vi "Begin.vi"(8 "error in":errorcluster) -> (0 "error out":errorcluster)   [LabVIEW 2015]
doc: "Called before other user functions, this VI is expected to open initial I/O refnums, load in file data, and do all program initialization. Notice that the <B>error out</B> terminal is simply used for data flow. Wiring it to other structures or subVIs ensures that this VI runs first."
uses:
  <vilib>/Rock Robotics/SystemInterfaces/DIO/FPGA_DIOPWMChannel.ctl
  <vilib>/Rock Robotics/WPI/SafetyOutput/WPI_SafetyOutputConfigMenu.ctl
  <vilib>/Rock Robotics/WPI/DriverStation/WPI_DriverStationRobotMode2.ctl
  <vilib>/Rock Robotics/WPI/Joystick/WPI_JoystickDeviceEnum.ctl
  <vilib>/Rock Robotics/SystemInterfaces/DIO/FPGA_DIOChannel.ctl
  <vilib>/Rock Robotics/SystemInterfaces/DIO/FPGA_DIORelayChannel.ctl
  <vilib>/Rock Robotics/WPI/Encoder/WPI_EncoderType.ctl
  <vilib>/Rock Robotics/WPI/Relay/WPI_RelayDirection.ctl
  <vilib>/Rock Robotics/SystemInterfaces/spilib/spi_bus.ctl
  <vilib>/Rock Robotics/WPI/RobotDrive/WPI_RobotDriveOpen2MotorWithVictor.vi
  Robot Global Data.vi
  <vilib>/Rock Robotics/Network Tables/NT Write String Array.vi
  <vilib>/Rock Robotics/WPI/Counter/WPI_CounterDigitalInputToDigitalSource.vi
  <vilib>/Rock Robotics/WPI/MotorControl/WPI_MotorControlOpen Victor.vi
  <vilib>/Rock Robotics/WPI/Gyro/WPI_GyroXRS450_SPI_Open.vi
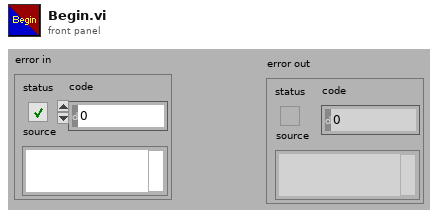
[diagram p1: front panel]
types:
  T1 = typedef "spi_bus.ctl" = enum16{"SPI On-Board, CS0", "SPI On-Board, CS1", "SPI On-Board, CS2", "SPI On-Board, CS3", "SPI MXP", "Invalid"}
  T2 = typedef "FPGA_DIOPWMChannel.ctl" = enum8{"PWM 0", "PWM 1", "PWM 2", "PWM 3", "PWM 4", "PWM 5", "PWM 6", "PWM 7", "PWM 8", "PWM 9", "PWM MXP 0", "PWM MXP 1", "PWM MXP 2", "PWM MXP 3", "PWM MXP 4", "PWM MXP 5", "PWM MXP 6", "PWM MXP 7", "PWM MXP 8", "PWM MXP 9", "Invalid"}
  T3 = typedef "WPI_RelayDirection.ctl" = enum16{"Both directions", "Forward only", "Reverse only"}
  T4 = typedef "FPGA_DIORelayChannel.ctl" = enum8{"Relay 0", "Relay 1", "Relay 2", "Relay 3", "Invalid"}
  T5 = typedef "FPGA_DIOChannel.ctl" = enum8{"DIO 0", "DIO 1", "DIO 2", "DIO 3", "DIO 4", "DIO 5", "DIO 6", "DIO 7", "DIO 8", "DIO 9", "DIO MXP 0", "DIO MXP 1", "DIO MXP 2", "DIO MXP 3", "DIO MXP 4", "DIO MXP 5", "DIO MXP 6", "DIO MXP 7", "DIO MXP 8", "DIO MXP 9", "DIO MXP 10", "DIO MXP 11", "DIO MXP 12", "DIO MXP 13", "DIO MXP 14", "DIO MXP 15", "Invalid"}
  T6 = typedef "WPI_EncoderType.ctl" = enum16{"1x", "2x", "4x"}
  T7 = typedef "WPI_JoystickDeviceEnum.ctl" = enum16{"USB 0", "USB 1", "USB 2", "USB 3", "USB 4", "USB 5"}
  T8 = typedef "WPI_SafetyOutputConfigMenu.ctl" = enum16{"Enable", "Disable"}
  T9 = typedef "WPI_DriverStationRobotMode2.ctl" = enum16{"Autonomous Disabled", "Autonomous Enabled", "Teleop Disabled", "Teleop Enabled", "Disconnected", "Finish", "Test Disabled", "Test Enabled", "Emergency Stopped"}
  T10 = typedef "WPI_MotorControlDeviceRef.ctl" = cluster{"DeviceStatus":errorcluster, "Type":T11, "PWM":cluster{"PWM Channel":T2, "DeadBand":T12}, "CAN":cluster{"Device Number":u8, "Control Mode":T13, "Semaphore":T14, "Max Vout":dbl, "TalonSRX Control Mode":T15}, "Invert":bool}
  T11 = typedef "WPI_MotorControlType.ctl" = enum16{"PWM", "CAN", "CANTalonSRX"}
  T12 = typedef "WPI_PWMDeadband.ctl" = cluster{"Name":string, "maxPositivePwm":i32, "minPositivePwm":i32, "centerPwm":i32, "maxNegativePwm":i32, "minNegativePwm":i32, "angularRange":u16}
  T13 = typedef "WPI_CANJaguar_ControlMode.ctl" = enum8{"Percent VBus", "Current", "Speed", "Position", "Voltage"}
  T14 = typedef "Semaphore RefNum" = refnum<k1>
  T15 = typedef "WPI_CANTalonSRX_APIControlMode.ctl" = enum8{"Percent VBus", "Speed", "Position", "Slave", "Unchanged / Invalid", "Voltage Compensation", "Current", "Motion Profile"}
  T16 = typedef "WPI_JoystickDevRef.ctl" = cluster{"Device":T7}
  T17 = typedef "WPI_RobotDriveDevRef.ctl" = cluster{"DevStatus":errorcluster, "Motors[]":T10[], "Square Inputs":bool, "Max Output":dbl}
  T18 = typedef "WPI_RelayDevRef.ctl" = cluster{"DevStatus":errorcluster, "Relay Channel":T4, "Relay Direction":T3}
  T19 = typedef "WPI_DigitalInputDevRef.ctl" = cluster{"DevStatus":errorcluster, "DIO Channel":T5}
  T20 = typedef "FPGA_CounterEncoderSourceConvertionLVSourceType.ctl" = cluster{"DevStatus":errorcluster, "AnalogTriggerMode?":bool, "DigitalMode":cluster{"DIO Channel":T21}, "AnalogTriggerMode":cluster{"AnalogTriggerIndex":T22, "OutputType":T23}}
  T21 = typedef "FPGA_DIODigitalSourceChannel.ctl" = enum8{"DIO 0", "DIO 1", "DIO 2", "DIO 3", "DIO 4", "DIO 5", "DIO 6", "DIO 7", "DIO 8", "DIO 9", "DIO MXP 0", "DIO MXP 1", "DIO MXP 2", "DIO MXP 3", "DIO MXP 4", "DIO MXP 5", "DIO MXP 6", "DIO MXP 7", "DIO MXP 8", "DIO MXP 9", "DIO MXP 10", "DIO MXP 11", "DIO MXP 12", "DIO MXP 13", "DIO MXP 14", "DIO MXP 15", "Disabled"}
  T22 = typedef "FPGA_AnalogTriggerIndex.ctl" = enum8{"Trig 0", "Trig 1", "Trig 2", "Trig 3", "Trig 4", "Trig 5", "Trig 6", "Trig 7", "Invalid"}
  T23 = typedef "FPGA_AnalogTriggerOutType.ctl" = enum16{"InWindow", "TriggerState", "Rising", "Falling"}
  T24 = typedef "WPI_EncoderDevRef.ctl" = cluster{"DevStatus":errorcluster, "EncoderIndex":T25, "CounterIndex":T26, "DistancePerCount":dbl, "Decoding Type":T6}
  T25 = typedef "FPGA_EncoderIdx.ctl" = enum8{"Enc 0", "Enc 1", "Enc 2", "Enc 3", "Enc 4", "Enc 5", "Enc 6", "Enc 7", "Invalid"}
  T26 = typedef "FPGA_CounterCtrSystemIndex.ctl" = enum8{"Ctr 0", "Ctr 1", "Ctr 2", "Ctr 3", "Ctr 4", "Ctr 5", "Ctr 6", "Ctr 7", "Invalid"}
  T27 = typedef "WPI_GyroDevRef.ctl" = cluster{"DevStatus":errorcluster, "Analog Channel":T28, "Offset":dbl, "Gain (VoltsPerDegree/Second)":dbl, "Gyro Type":enum16{"Analog", "XRS450"}, "Handle":i32, "SPI Bus":T1, "Device Found":bool, "Sample Rate":dbl, "Calibrate On Open":bool}
  T28 = typedef "FPGA_AIChannel.ctl" = enum8{"AI 0", "AI 1", "AI 2", "AI 3", "AI MXP 0", "AI MXP 1", "AI MXP 2", "AI MXP 3", "Invalid"}
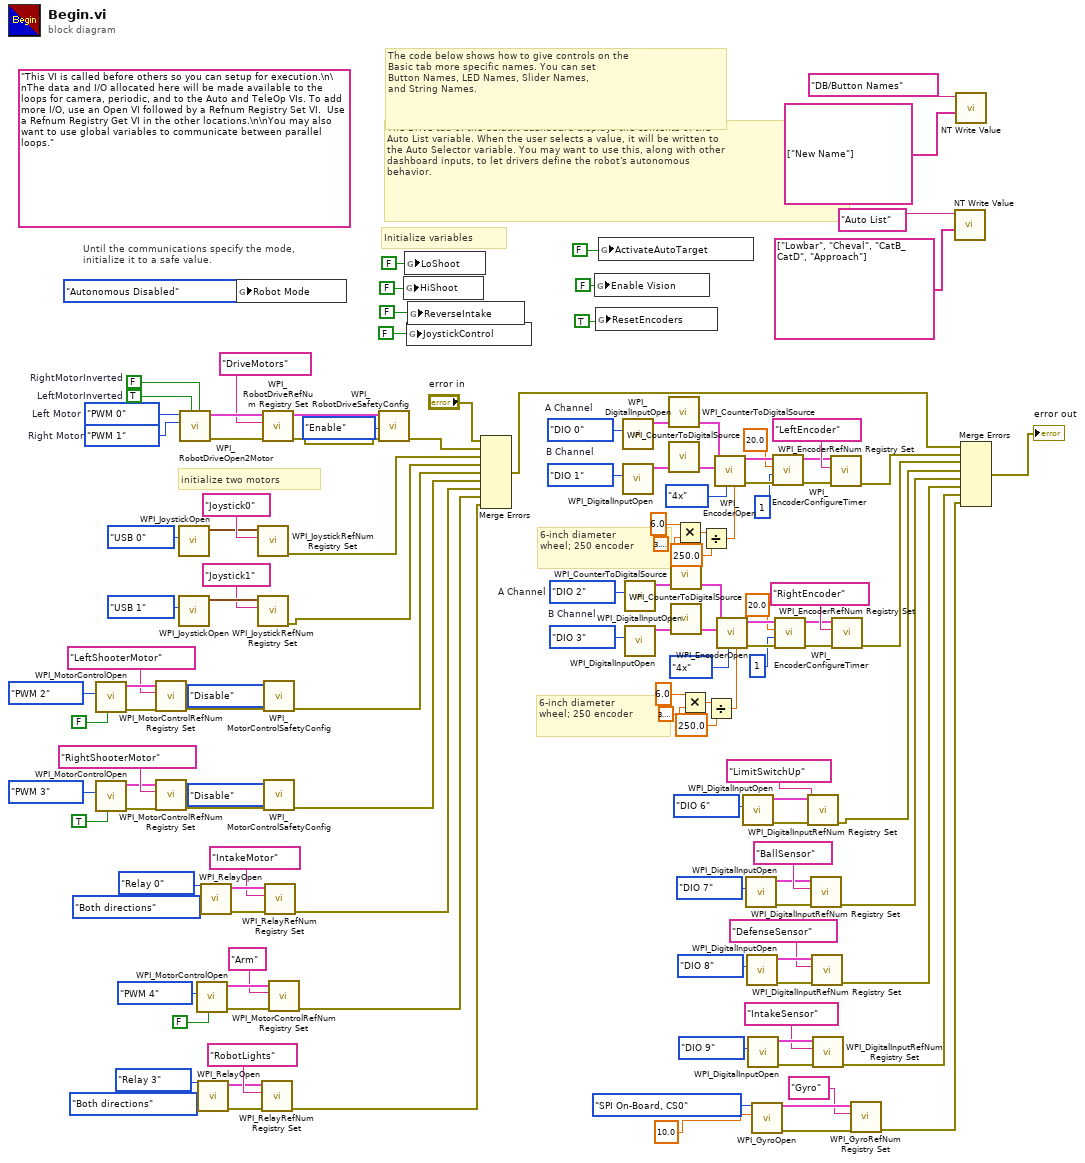
[diagram p0: block diagram]
diagram:
  w109 = FPGA_DIOChannel."DIO 3"  # B Channel
  w108 = FPGA_DIOChannel."DIO 2"  # A Channel
  w116 = FPGA_DIOChannel."DIO 1"  # B Channel
  w115 = FPGA_DIOChannel."DIO 0"  # A Channel
  (unwired) "This VI is called before others so you can setup for execution.\n\nThe data and I/O allocated here will be made available to the loops for camera, periodic, and to the Auto and TeleOp VIs. To add more I/O, use an Open VI followed by a Refnum Registry Set VI.  Use a Refnum Registry Get VI in the other locations.\n\nYou may also want to use global variables to communicate between parallel loops."
  w130 = FPGA_DIOPWMChannel."PWM 1"  # Right Motor
  w131 = FPGA_DIOPWMChannel."PWM 0"  # Left Motor
  w135 = TRUE  # LeftMotorInverted
  w136 = FALSE  # RightMotorInverted
  # "Initialize variables"
  # "6-inch diameter\nwheel; 250 encoder"
  # "6-inch diameter\nwheel; 250 encoder"
  # "The Drive tab of the default dashboard displays the contents of the\nAuto List variable. When the user selects a value, it will be written to\nthe Auto Selector variable. You may want to use this, along with other\ndashboard inputs, to let drivers define the robot's autonomous\nbehavior."
  # "The code below shows how to give controls on the\nBasic tab more specific names. You can set\nButton Names, LED Names, Slider Names,\nand String Names."
  # "Until the communications specify the mode,\ninitialize it to a safe value."
  # "initialize two motors"
  n1 = call-poly <vilib>:"WPI_MotorControlOpen.vi"("Invert"=FALSE, "PWM Channel"=FPGA_DIOPWMChannel."PWM 2") -> ("error out"=w100:errorcluster, "MotorControlDeviceRef"=w99:T10)  [unwired: 8 in]
  n2 = call-poly <vilib>:"WPI_MotorControlOpen.vi"("Invert"=TRUE, "PWM Channel"=FPGA_DIOPWMChannel."PWM 3") -> ("error out"=w89:errorcluster, "MotorControlDeviceRef"=w90:T10)  [unwired: 8 in]
  n3 = call <vilib>:"WPI_MotorControlRefNum Registry Set.vi"("error in (no error)"=w100, "refnum name"="LeftShooterMotor", "MotorControlDevRef"=w99) -> ("error out"=w96:errorcluster, "MotorControlDevRef"=w97:T10)  [unwired: 7 in]
  n4 = call <vilib>:"WPI_MotorControlRefNum Registry Set.vi"("error in (no error)"=w89, "refnum name"="RightShooterMotor", "MotorControlDevRef"=w90) -> ("error out"=w93:errorcluster, "MotorControlDevRef"=w92:T10)  [unwired: 7 in]
  n5 = call <vilib>:"WPI_JoystickOpen.vi"("JoystickDevice"=WPI_JoystickDeviceEnum."USB 0") -> ("JoystickDevRef"=w125:T16)  [unwired: 10 in]
  n6 = call <vilib>:"WPI_JoystickOpen.vi"("JoystickDevice"=WPI_JoystickDeviceEnum."USB 1") -> ("JoystickDevRef"=w68:T16)  [unwired: 10 in]
  n7 = call-poly <vilib>:"WPI_RobotDriveOpen2Motor.vi"("Right Motor Inverted"=w136, "Left Motor Inverted"=w135, "Right Motor"=w130, "Left Motor"=w131) -> ("error out"=w132:errorcluster, "RobotDriveDevRef"=w134:T17)  [unwired: 1 in, 5 out]
  n8 = call-poly <vilib>:"WPI_MotorControlOpen.vi"("Invert"=FALSE, "PWM Channel"=FPGA_DIOPWMChannel."PWM 4") -> ("error out"=w9:errorcluster, "MotorControlDeviceRef"=w11:T10)  [unwired: 8 in]
  n9 = call <vilib>:"WPI_RelayOpen.vi"("Relay Direction"=WPI_RelayDirection."Both directions", "Relay Channel"=FPGA_DIORelayChannel."Relay 3") -> ("error out"=w19:errorcluster, "RelayDevRef"=w20:T18)  [unwired: 8 in]
  n10 = call <vilib>:"WPI_RelayOpen.vi"("Relay Direction"=WPI_RelayDirection."Both directions", "Relay Channel"=FPGA_DIORelayChannel."Relay 0") -> ("error out"=w75:errorcluster, "RelayDevRef"=w74:T18)  [unwired: 8 in]
  n11 = global write "Robot Global Data.vi" "Robot Mode"(WPI_DriverStationRobotMode2."Autonomous Disabled" ("Robot Mode")) -> ()
  n12 = call <vilib>:"WPI_JoystickRefNum Registry Set.vi"("refnum name"="Joystick0", "JoystickDevRef"=w125) -> ("error out"=w117:errorcluster)  [unwired: 8 in, 1 out]
  n13 = call <vilib>:"WPI_JoystickRefNum Registry Set.vi"("refnum name"="Joystick1", "JoystickDevRef"=w68) -> ("error out"=w64:errorcluster)  [unwired: 8 in, 1 out]
  n14 = call <vilib>:"WPI_RelayRefNum Registry Set.vi"("error in (no error)"=w19, "refnum name"="RobotLights", "RelayDevRef"=w20) -> ("error out"=w16:errorcluster)  [unwired: 7 in, 1 out]
  n15 = call <vilib>:"WPI_RobotDriveRefNum Registry Set.vi"("error in (no error)"=w132, "refnum name"="DriveMotors", "RobotDriveDevRef"=w134) -> ("error out"=w119:errorcluster, "RobotDriveDevRef"=w129:T17)  [unwired: 1 in, 6 out]
  n16 = call <vilib>:"WPI_MotorControlSafetyConfig.vi"("error in (no error)"=w96, "mode"=WPI_SafetyOutputConfigMenu."Disable", "MotorControlDevRef"=w97) -> ("error out"=w65:errorcluster)  [unwired: 7 in, 1 out]
  n17 = call <vilib>:"WPI_MotorControlSafetyConfig.vi"("error in (no error)"=w93, "mode"=WPI_SafetyOutputConfigMenu."Disable", "MotorControlDevRef"=w92) -> ("error out"=w66:errorcluster)  [unwired: 7 in, 1 out]
  n18 = call <vilib>:"WPI_RelayRefNum Registry Set.vi"("error in (no error)"=w75, "refnum name"="IntakeMotor", "RelayDevRef"=w74) -> ("error out"=w32:errorcluster)  [unwired: 7 in, 1 out]
  n19 = call <vilib>:"WPI_MotorControlRefNum Registry Set.vi"("error in (no error)"=w9, "refnum name"="Arm", "MotorControlDevRef"=w11) -> ("error out"=w12:errorcluster)  [unwired: 7 in, 1 out]
  n20 = call <vilib>:"WPI_RobotDriveSafetyConfig.vi"("error in (no error)"=w119, "mode"=WPI_SafetyOutputConfigMenu."Enable", "RobotDriveDevRef"=w129) -> ("error out"=w118:errorcluster)  [unwired: 7 in, 1 out]
  n21 = global write "Robot Global Data.vi" "HiShoot"(FALSE ("Shoot")) -> ()
  n22 = global write "Robot Global Data.vi" "LoShoot"(FALSE ("Shoot")) -> ()
  n23 = global write "Robot Global Data.vi" "JoystickControl"(FALSE) -> ()
  n24 = global write "Robot Global Data.vi" "ReverseIntake"(FALSE ("Shoot")) -> ()
  n25 = Merge Errors("error in", w118, w117, w64, w65, w66, w32, w12, w16) -> (w72:errorcluster)
  n26 = global write "Robot Global Data.vi" "Enable Vision"(FALSE) -> ()
  n27 = global write "Robot Global Data.vi" "ResetEncoders"(TRUE) -> ()
  n28 = global write "Robot Global Data.vi" "ActivateAutoTarget"(FALSE ("ActiveTarget")) -> ()
  n29 = call <vilib>:"WPI_DigitalInputOpen.vi"("DIO Channel"=w115) -> ("DigitalInputDevRef"=w112:T19)  [unwired: 1 in, 9 out]
  n30 = call <vilib>:"WPI_DigitalInputOpen.vi"("DIO Channel"=w116) -> ("DigitalInputDevRef"=w113:T19)  [unwired: 1 in, 9 out]
  n31 = call <vilib>:"WPI_DigitalInputOpen.vi"("DIO Channel"=w108) -> ("DigitalInputDevRef"=w105:T19)  [unwired: 1 in, 9 out]
  n32 = call <vilib>:"WPI_DigitalInputOpen.vi"("DIO Channel"=w109) -> ("DigitalInputDevRef"=w106:T19)  [unwired: 1 in, 9 out]
  n33 = call-poly <vilib>:"WPI_CounterToDigitalSource.vi"("DigitalInputDevRef"=w112) -> ("Digital Source"=w111:T20)  [unwired: 6 out]
  n34 = call-poly <vilib>:"WPI_CounterToDigitalSource.vi"("DigitalInputDevRef"=w113) -> ("Digital Source"=w114:T20)  [unwired: 6 out]
  n35 = call-poly <vilib>:"WPI_CounterToDigitalSource.vi"("DigitalInputDevRef"=w105) -> ("Digital Source"=w104:T20)  [unwired: 6 out]
  n36 = call-poly <vilib>:"WPI_CounterToDigitalSource.vi"("DigitalInputDevRef"=w106) -> ("Digital Source"=w107:T20)  [unwired: 6 out]
  n37 = Multiply(x=6.0, y=3.141592653589793) -> (x*y=w60:dbl)
  n38 = Multiply(x=6.0, y=3.141592653589793) -> (x*y=w56:dbl)
  n39 = Divide(x=w60, y=250.0) -> (x/y=w58:dbl)
  n40 = Divide(x=w56, y=250.0) -> (x/y=w53:dbl)
  n41 = call <vilib>:"WPI_EncoderOpen.vi"("DistancePerCount"=w58, "Decoding Type"=WPI_EncoderType."4x", "BSource"=w114, "ASource"=w111) -> ("error out"=w41:errorcluster, "EncoderDevRef"=w42:T24)  [unwired: 4 in, 2 out]
  n42 = call <vilib>:"WPI_EncoderOpen.vi"("DistancePerCount"=w53, "Decoding Type"=WPI_EncoderType."4x", "BSource"=w107, "ASource"=w104) -> ("error out"=w46:errorcluster, "EncoderDevRef"=w45:T24)  [unwired: 4 in, 2 out]
  n43 = call <vilib>:"WPI_DigitalInputOpen.vi"("DIO Channel"=FPGA_DIOChannel."DIO 6") -> ("error out"=w27:errorcluster, "DigitalInputDevRef"=w28:T19)  [unwired: 9 in]
  n44 = call <vilib>:"WPI_DigitalInputOpen.vi"("DIO Channel"=FPGA_DIOChannel."DIO 7") -> ("error out"=w35:errorcluster, "DigitalInputDevRef"=w34:T19)  [unwired: 9 in]
  n45 = call <vilib>:"WPI_DigitalInputOpen.vi"("DIO Channel"=FPGA_DIOChannel."DIO 8") -> ("error out"=w82:errorcluster, "DigitalInputDevRef"=w83:T19)  [unwired: 9 in]
  n46 = call <vilib>:"WPI_DigitalInputOpen.vi"("DIO Channel"=FPGA_DIOChannel."DIO 9") -> ("error out"=w80:errorcluster, "DigitalInputDevRef"=w81:T19)  [unwired: 9 in]
  n47 = call-poly <vilib>:"WPI_GyroOpen.vi"("Sample Rate (ms)"=10.0, "SPI Bus"=spi_bus."SPI On-Board, CS0") -> ("error out"=w2:errorcluster, "GyroDevRef"=w4:T27)  [unwired: 8 in]
  n48 = call <vilib>:"WPI_EncoderConfigureTimer.vi"("error in (no error)"=w41, "Number Samples to Average"=u8 1, "Minimum Rate"=20.0, "EncoderDevRef"=w42) -> ("error out"=w48:errorcluster, "EncoderDevRef"=w47:T24)  [unwired: 6 in]
  n49 = call <vilib>:"WPI_EncoderConfigureTimer.vi"("error in (no error)"=w46, "Number Samples to Average"=u8 1, "Minimum Rate"=20.0, "EncoderDevRef"=w45) -> ("error out"=w43:errorcluster, "EncoderDevRef"=w44:T24)  [unwired: 6 in]
  n50 = call <vilib>:"WPI_DigitalInputRefNum Registry Set.vi"("error in (no error)"=w27, "refnum name"="LimitSwitchUp", "DigitalInputDevRef"=w28) -> ("error out"=w22:errorcluster)  [unwired: 7 in, 1 out]
  n51 = call <vilib>:"WPI_DigitalInputRefNum Registry Set.vi"("error in (no error)"=w35, "refnum name"="BallSensor", "DigitalInputDevRef"=w34) -> ("error out"=w23:errorcluster)  [unwired: 7 in, 1 out]
  n52 = call <vilib>:"WPI_DigitalInputRefNum Registry Set.vi"("error in (no error)"=w82, "refnum name"="DefenseSensor", "DigitalInputDevRef"=w83) -> ("error out"=w24:errorcluster)  [unwired: 7 in, 1 out]
  n53 = call <vilib>:"WPI_DigitalInputRefNum Registry Set.vi"("error in (no error)"=w80, "refnum name"="IntakeSensor", "DigitalInputDevRef"=w81) -> ("error out"=w25:errorcluster)  [unwired: 7 in, 1 out]
  n54 = call <vilib>:"WPI_EncoderRefNum Registry Set.vi"("error in (no error)"=w48, "refnum name"="LeftEncoder", "EncoderDevRef"=w47) -> ("error out"=w71:errorcluster)  [unwired: 7 in, 1 out]
  n55 = call <vilib>:"WPI_EncoderRefNum Registry Set.vi"("error in (no error)"=w43, "refnum name"="RightEncoder", "EncoderDevRef"=w44) -> ("error out"=w70:errorcluster)  [unwired: 7 in, 1 out]
  n56 = call <vilib>:"WPI_GyroRefNum Registry Set.vi"("error in (no error)"=w2, "refnum name"="Gyro", "GyroDevRef"=w4) -> ("error out"=w1:errorcluster)  [unwired: 7 in, 1 out]
  n57 = call-poly <vilib>:"NT Write Value.vi"("String Array"=string[] ["Lowbar", "Cheval", "CatB_CatD", "Approach"], "Name"="Auto List") -> ()  [unwired: 9 in, 1 out]
  n58 = call-poly <vilib>:"NT Write Value.vi"("String Array"=string[] ["New Name"], "Name"="DB/Button Names") -> ()  [unwired: 9 in, 1 out]
  n59 = Merge Errors(w72, w71, w70, w22, w23, w24, w25, w1) -> (→"error out":errorcluster)
